vi "Main.vi"() -> ()   [LabVIEW 2010]
panel:
  out "*(type *) &x":u8
  out "unsigned 16bit integer":u16
  in  "Sample Configuration":T1(ring)
  out "Bytes Written 3":u32
  out "FT_Status 3":u32(ring) items=["FT_OK", "FT_INVALID_HANDLE", "FT_DEVICE_NOT_FOUND", "FT_DEVICE_NOT_OPENED", "FT_IO_ERROR", "FT_INSUFFICIENT_RESOURCES", "FT_INVALID_PARAMETER", "FT_INVALID_BAUD_RATE", "FT_DEVICE_NOT_OPENED_FOR_ERASE", "FT_DEVICE_NOT_OPENED_FOR_WRITE", "FT_FAILED_TO_WRITE_DEVICE", "FT_EEPROM_READ_FAILED", "FT_EEPROM_WRITE_FAILED", "FT_EEPROM_ERASE_FAILED", "FT_EEPROM_NOT_PRESENT", "FT_EEPROM_NOT_PROGRAMMED", "FT_INVALID_ARGS", "FT_NOT_SUPPORTED", "FT_OTHER_ERROR"]
  in  "Sampling Period (us)":i32=10 format="%.d"
  in  "Number of Samples":i32=1024
  in  "StopSampling":bool
  in  "StartSampling":bool
  out "XY Graph":cluster{i32[], dbl[]}[](graph)
  in  "Current Scale":enum8{"100 mA", "200 mA", "500 mA", "1 A"}(ring)
  in  "SetCurrentScale":bool
  in  "Gain":i16=700
  out "Bytes Written 2":u32
  out "FT_Status 2":u32(ring) items=["FT_OK", "FT_INVALID_HANDLE", "FT_DEVICE_NOT_FOUND", "FT_DEVICE_NOT_OPENED", "FT_IO_ERROR", "FT_INSUFFICIENT_RESOURCES", "FT_INVALID_PARAMETER", "FT_INVALID_BAUD_RATE", "FT_DEVICE_NOT_OPENED_FOR_ERASE", "FT_DEVICE_NOT_OPENED_FOR_WRITE", "FT_FAILED_TO_WRITE_DEVICE", "FT_EEPROM_READ_FAILED", "FT_EEPROM_WRITE_FAILED", "FT_EEPROM_ERASE_FAILED", "FT_EEPROM_NOT_PRESENT", "FT_EEPROM_NOT_PROGRAMMED", "FT_INVALID_ARGS", "FT_NOT_SUPPORTED", "FT_OTHER_ERROR"]
  in  "SetGain":bool
  in  "ChangeFrequency":bool
  in  "Frequency 3 (Hz)":i32=99000
  in  "Phase 3(º)":T2(ring)
  in  "Frequency 2 (Hz)":i32=99000
  in  "Phase 2 (º)":T2(ring)
  in  "Phase 1 (º)":T2(ring)
  in  "Frequency 1 (Hz)":i32=100000 format="%.d"
  out "ChB Data":i16[](array[numeric]) format="%x"
  out "ChA Data":i16[](array[numeric]) format="%x"
  out "Read Data":u8[](array[numeric]) format="%x"
  out "size(s)":i32
  out "FT_Status":u32(ring) items=["FT_OK", "FT_INVALID_HANDLE", "FT_DEVICE_NOT_FOUND", "FT_DEVICE_NOT_OPENED", "FT_IO_ERROR", "FT_INSUFFICIENT_RESOURCES", "FT_INVALID_PARAMETER", "FT_INVALID_BAUD_RATE", "FT_DEVICE_NOT_OPENED_FOR_ERASE", "FT_DEVICE_NOT_OPENED_FOR_WRITE", "FT_FAILED_TO_WRITE_DEVICE", "FT_EEPROM_READ_FAILED", "FT_EEPROM_WRITE_FAILED", "FT_EEPROM_ERASE_FAILED", "FT_EEPROM_NOT_PRESENT", "FT_EEPROM_NOT_PROGRAMMED", "FT_INVALID_ARGS", "FT_NOT_SUPPORTED", "FT_OTHER_ERROR"]
  in  "Stop Program":bool
  in  "Read":bool
  out "Bytes Waiting":u32
  out "Bytes Read":u32
  out "Description ChB":string
  out "Description ChA":string
  out "Handle ChB 2":u32
  out "Handle ChA":u32
  out "Status":bool
  in  "ChA Write Buffer":string="\u0017"
  out "Bytes Written":u32
  # "DDS Change Frequency"
  # "Set Amplification Gain"
  # "Set Probe Current Scale"
  # "Start Sampling"
  # "Configuration and Setup"
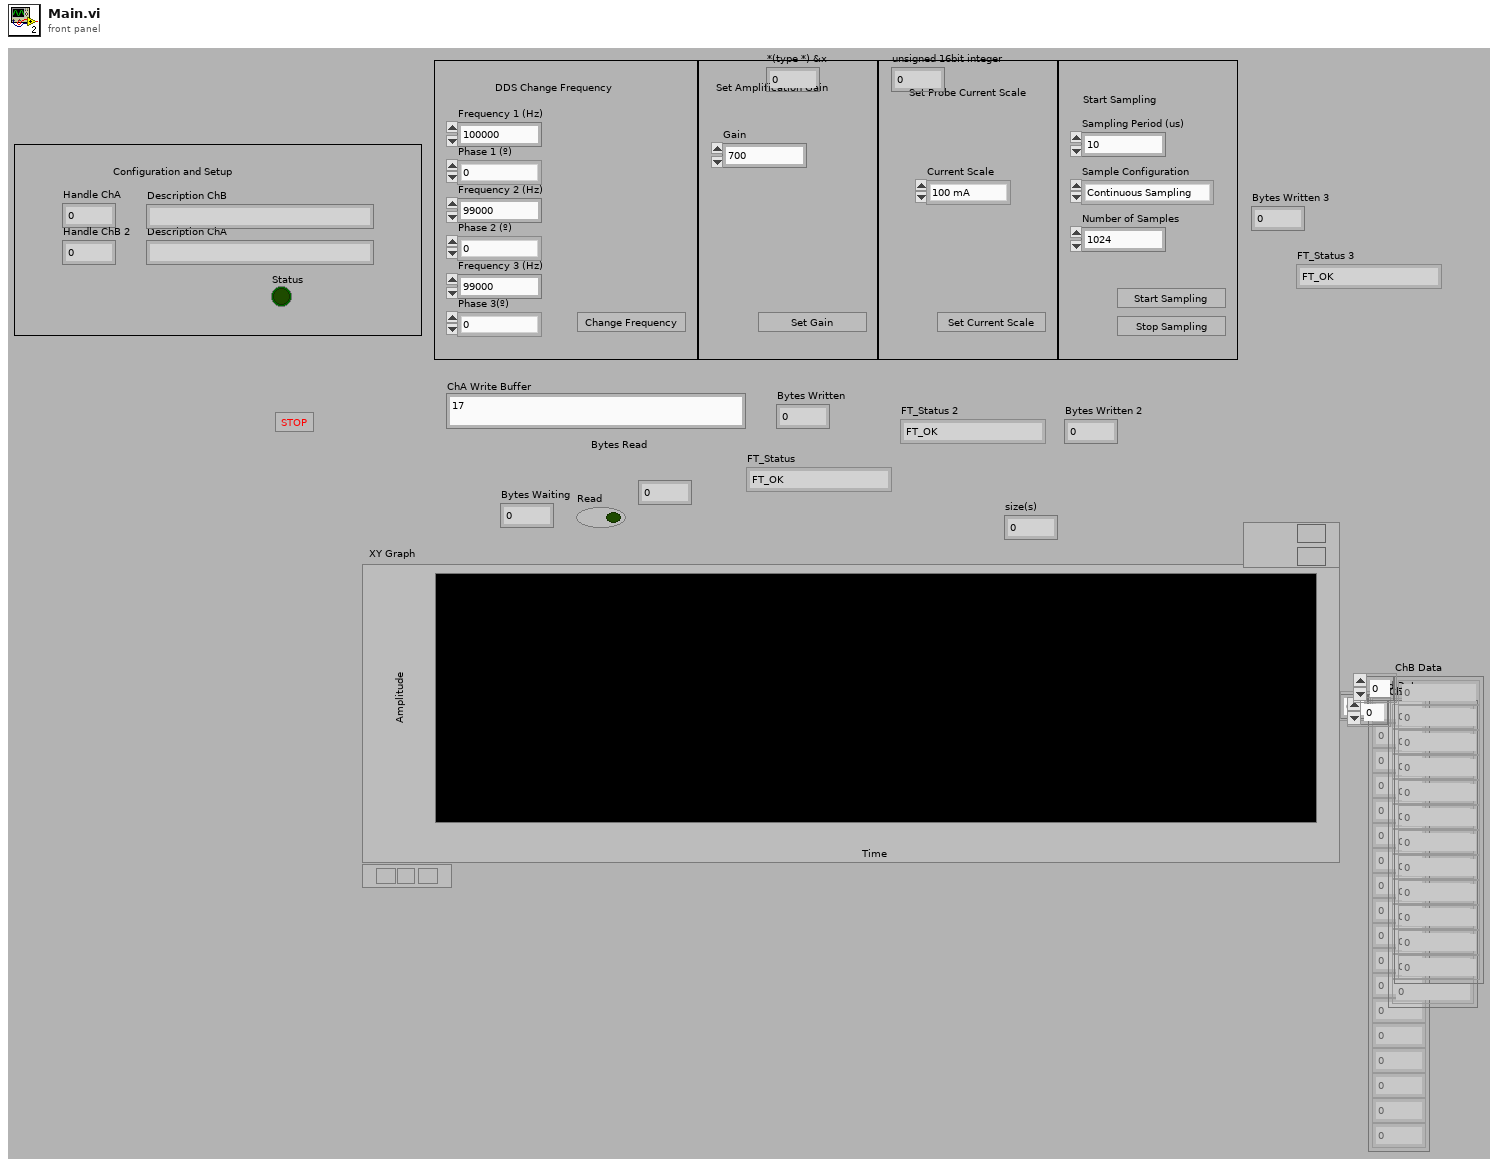
[diagram p1: front panel]
types:
  T1 = enum8{"Continuous Sampling", "Single Acquisiton"}
  T2 = enum8{"0", "11.25", "22.5", "33.75", "45", "56.25", "67.5", "78.75", "90", "101.25", "112.5", "123.75", "135", "146.25", "157.5", "168.75", "180", "191.25", "202.5", "213.75", "225", "236.25", "247.5", "258.75", "270", "281.25", "292.5", "303.75", "315", "326.25", "337.5", "348.75", "360"}
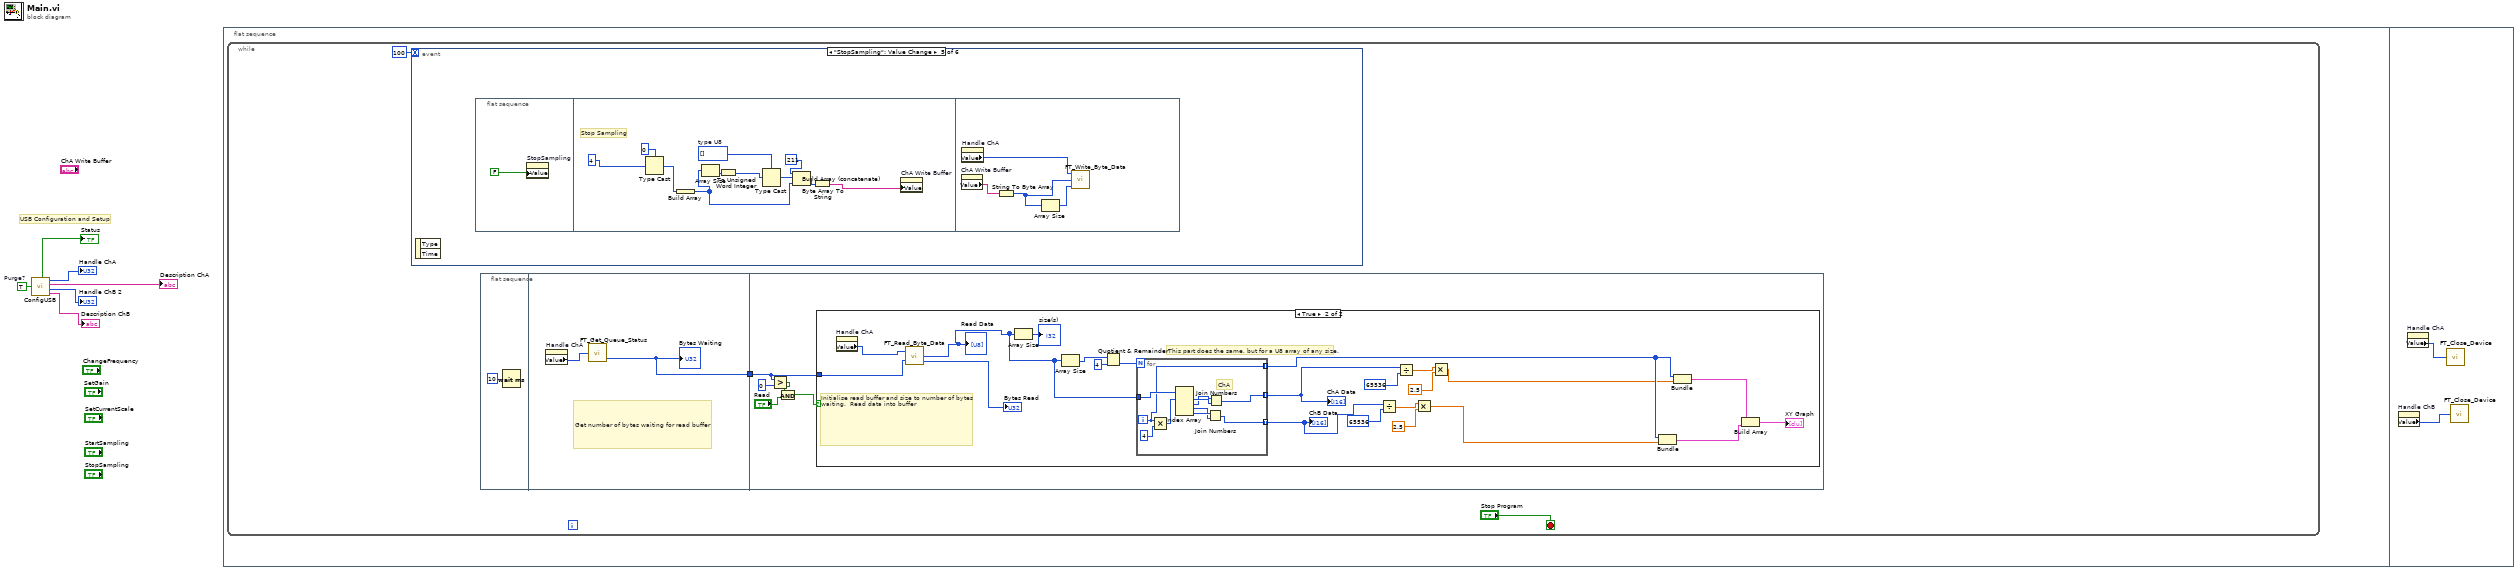
[diagram p0: block diagram]
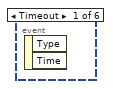
[diagram p2: hidden frame]
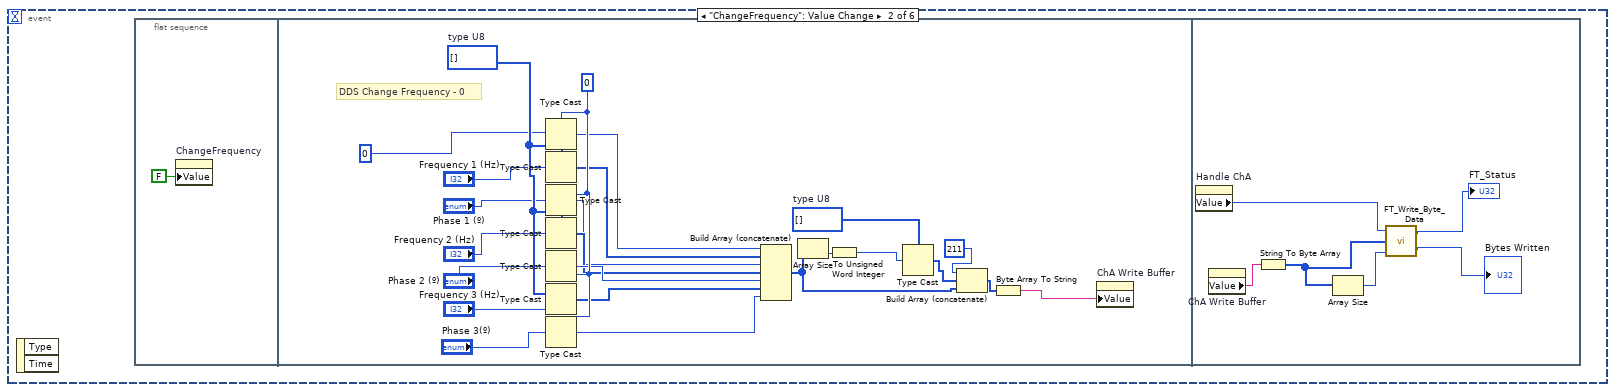
[diagram p3: hidden frame]
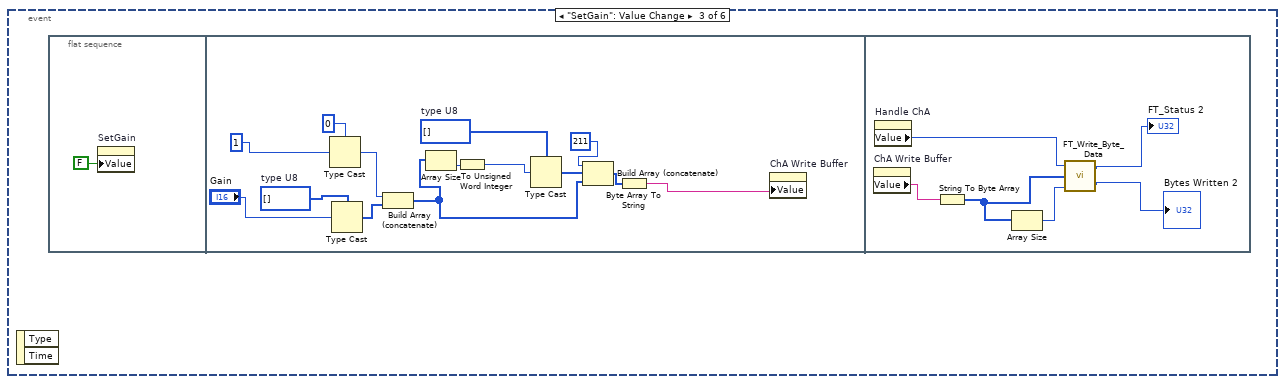
[diagram p4: hidden frame]
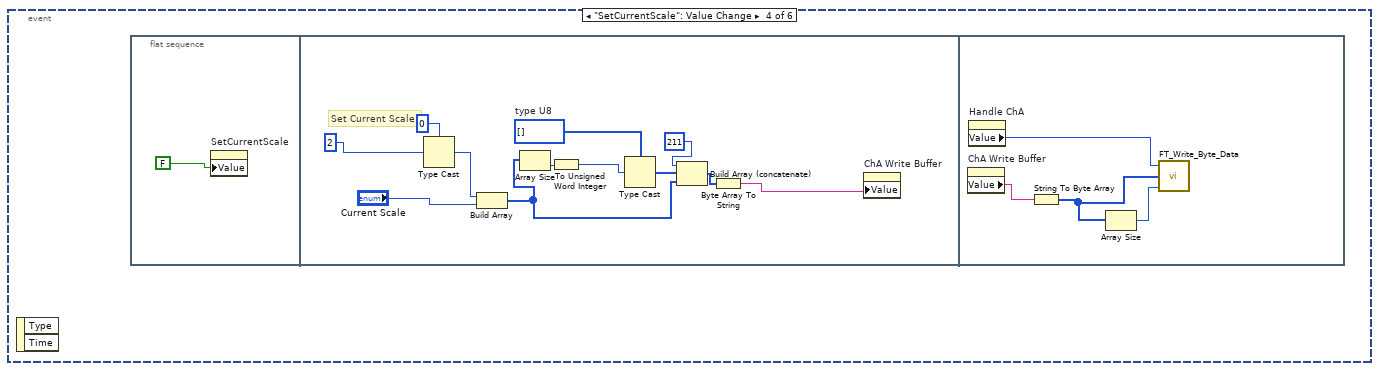
[diagram p5: hidden frame]
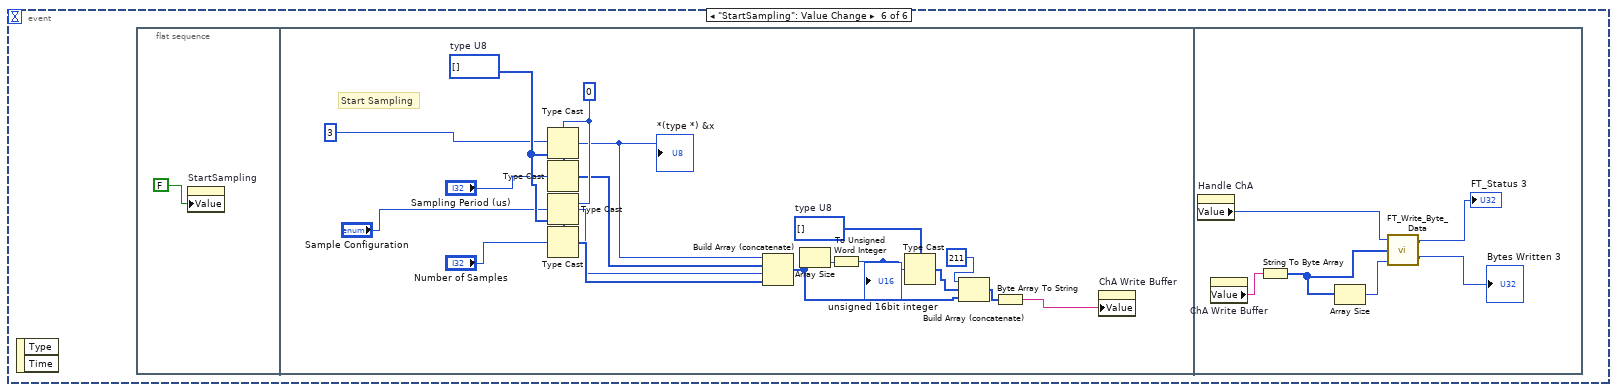
[diagram p6: hidden frame]
diagram:
  w5 = TRUE  # Purge?
  # "USB Configuration and Setup"
  n1 = call "ConfigUSB.vi"("Purge?"=w5) -> ("Status"=→"Status":bool, "Handle ChA"=→"Handle ChA":u32, "Description ChA"=→"Description ChA":string, "Handle ChB 2"=→"Handle ChB 2":u32, "Description ChB"=→"Description ChB":string)  [unwired: 5 in]
  n2 = flat-sequence {
    frame #0 {
      n3 = while {
        stop <- "Stop Program" stop-if-true
        n4 = event shown="[4] \"StopSampling\": Value Change" {
          selector: _ -> [_ _ _ _ _ _]
          dyn-events: _ -> [_ _ _ _ _ _]
          timeout: 100 -> [_ _ _ _ _ _]
          event Timeout {
            n5 = event-data() -> ()  [unwired: 1 in, 2 out]
          }
          event "ChangeFrequency": Value Change {
            n6 = event-data() -> ()  [unwired: 1 in, 2 out]
            n7 = flat-sequence {
              frame #0 {
                n8 = property on="ChangeFrequency" class="Bool (strict)"("Value"=FALSE ("ChangeFrequency")) -> ()  [unwired: 2 in, 2 out]
              }
              frame #1 {
                w32 = u8[] []  # type U8
                w29 = u8 0
                w25 = u8[] []  # type U8
                # "DDS Change Frequency - 0"
                n9 = Type Cast(type=w29, x=0) -> (*(type *) &x=w18:u8)
                n10 = Type Cast(type=w25, x="Frequency 1 (Hz)") -> (*(type *) &x=w19:u8[])
                n11 = Type Cast(type=w29, x="Phase 1 (º)") -> (*(type *) &x=w20:u8)
                n12 = Type Cast(type=w25, x="Frequency 2 (Hz)") -> (*(type *) &x=w21:u8[])
                n13 = Type Cast(type=w29, x="Phase 2 (º)") -> (*(type *) &x=w22:u8)
                n14 = Type Cast(type=w25, x="Frequency 3 (Hz)") -> (*(type *) &x=w23:u8[])
                n15 = Type Cast(type=w29, x="Phase 3(º)") -> (*(type *) &x=w24:u8)
                n16 = Build Array (concatenate)(w18, w19, w20, w21, w22, w23, w24) -> (w31:u8[])
                n17 = Array Size(array=w31) -> (size(s)=w30:i32)
                n18 = To Unsigned Word Integer(number=w30) -> (unsigned 16bit integer=w34:u16)
                n19 = Type Cast(type=w32, x=w34) -> (*(type *) &x=w33:u8[])
                n20 = Build Array (concatenate)(u8 211, w33, w31) -> (w27:u8[])
                n21 = Byte Array To String(unsigned byte array=w27) -> (string=w28:string)
                n22 = property on="ChA Write Buffer" class="Str"("Value"=w28) -> ()  [unwired: 2 in, 2 out]
              }
              frame #2 {
                n23 = property on="Handle ChA" class="DigNum (strict)"() -> ("Value"=w38:u32)  [unwired: 2 in, 2 out]
                n24 = property on="ChA Write Buffer" class="Str"() -> ("Value"=w35:string)  [unwired: 2 in, 2 out]
                n25 = String To Byte Array(string=w35) -> (unsigned byte array=w37:u8[])
                n26 = Array Size(array=w37) -> (size(s)=w36:i32)
                n27 = call "FT_Write_Byte_Data.vi"("Bytes To Write"=w36, "Buffer"=w37, "Handle"=w38) -> ("Bytes Written"=→"Bytes Written":u32, "FT_Status"=→"FT_Status":u32)
              }
            }
          }
          event "SetGain": Value Change {
            n28 = event-data() -> ()  [unwired: 1 in, 2 out]
            n29 = flat-sequence {
              frame #0 {
                n30 = property on="SetGain" class="Bool (strict)"("Value"=FALSE ("SetGain")) -> ()  [unwired: 2 in, 2 out]
              }
              frame #1 {
                w55 = u8[] []  # type U8
                w52 = u8[] []  # type U8
                n31 = Type Cast(type=u8 0, x=u8 1) -> (*(type *) &x=w44:u8)
                n32 = Type Cast(type=w55, x="Gain") -> (*(type *) &x=w45:u8[])
                n33 = Build Array (concatenate)(w44, w45) -> (w43:u8[])
                n34 = Array Size(array=w43) -> (size(s)=w53:i32)
                n35 = To Unsigned Word Integer(number=w53) -> (unsigned 16bit integer=w51:u16)
                n36 = Type Cast(type=w52, x=w51) -> (*(type *) &x=w54:u8[])
                n37 = Build Array (concatenate)(u8 211, w54, w43) -> (w49:u8[])
                n38 = Byte Array To String(unsigned byte array=w49) -> (string=w48:string)
                n39 = property on="ChA Write Buffer" class="Str"("Value"=w48) -> ()  [unwired: 2 in, 2 out]
              }
              frame #2 {
                n40 = property on="ChA Write Buffer" class="Str"() -> ("Value"=w56:string)  [unwired: 2 in, 2 out]
                n41 = property on="Handle ChA" class="DigNum (strict)"() -> ("Value"=w59:u32)  [unwired: 2 in, 2 out]
                n42 = String To Byte Array(string=w56) -> (unsigned byte array=w60:u8[])
                n43 = Array Size(array=w60) -> (size(s)=w61:i32)
                n44 = call "FT_Write_Byte_Data.vi"("Bytes To Write"=w61, "Buffer"=w60, "Handle"=w59) -> ("Bytes Written"=→"Bytes Written 2":u32, "FT_Status"=→"FT_Status 2":u32)
              }
            }
          }
          event "SetCurrentScale": Value Change {
            n45 = event-data() -> ()  [unwired: 1 in, 2 out]
            n46 = flat-sequence {
              frame #0 {
                n47 = property on="SetCurrentScale" class="Bool (strict)"("Value"=FALSE ("SetGain")) -> ()  [unwired: 2 in, 2 out]
              }
              frame #1 {
                w72 = u8[] []  # type U8
                # "Set Current Scale"
                n48 = Type Cast(type=u8 0, x=u8 2) -> (*(type *) &x=w66:u8)
                n49 = Build Array(w66, "Current Scale") -> (w65:u8[])
                n50 = Array Size(array=w65) -> (size(s)=w73:i32)
                n51 = To Unsigned Word Integer(number=w73) -> (unsigned 16bit integer=w71:u16)
                n52 = Type Cast(type=w72, x=w71) -> (*(type *) &x=w74:u8[])
                n53 = Build Array (concatenate)(u8 211, w74, w65) -> (w69:u8[])
                n54 = Byte Array To String(unsigned byte array=w69) -> (string=w68:string)
                n55 = property on="ChA Write Buffer" class="Str"("Value"=w68) -> ()  [unwired: 2 in, 2 out]
              }
              frame #2 {
                n56 = property on="ChA Write Buffer" class="Str"() -> ("Value"=w75:string)  [unwired: 2 in, 2 out]
                n57 = property on="Handle ChA" class="DigNum (strict)"() -> ("Value"=w76:u32)  [unwired: 2 in, 2 out]
                n58 = String To Byte Array(string=w75) -> (unsigned byte array=w77:u8[])
                n59 = Array Size(array=w77) -> (size(s)=w78:i32)
                n60 = call "FT_Write_Byte_Data.vi"("Bytes To Write"=w78, "Buffer"=w77, "Handle"=w76) -> ()  [unwired: 2 out]
              }
            }
          }
          event "StopSampling": Value Change {
            n61 = event-data() -> ()  [unwired: 1 in, 2 out]
            n62 = flat-sequence {
              frame #0 {
                n63 = property on="StopSampling" class="Bool (strict)"("Value"=FALSE ("SetGain")) -> ()  [unwired: 2 in, 2 out]
              }
              frame #1 {
                w88 = u8[] []  # type U8
                # "Stop Sampling"
                n64 = Type Cast(type=u8 0, x=u8 4) -> (*(type *) &x=w82:u8)
                n65 = Build Array(w82) -> (w81:u8[])
                n66 = Array Size(array=w81) -> (size(s)=w89:i32)
                n67 = To Unsigned Word Integer(number=w89) -> (unsigned 16bit integer=w87:u16)
                n68 = Type Cast(type=w88, x=w87) -> (*(type *) &x=w90:u8[])
                n69 = Build Array (concatenate)(u8 211, w90, w81) -> (w85:u8[])
                n70 = Byte Array To String(unsigned byte array=w85) -> (string=w84:string)
                n71 = property on="ChA Write Buffer" class="Str"("Value"=w84) -> ()  [unwired: 2 in, 2 out]
              }
              frame #2 {
                n72 = property on="ChA Write Buffer" class="Str"() -> ("Value"=w91:string)  [unwired: 2 in, 2 out]
                n73 = property on="Handle ChA" class="DigNum (strict)"() -> ("Value"=w92:u32)  [unwired: 2 in, 2 out]
                n74 = String To Byte Array(string=w91) -> (unsigned byte array=w93:u8[])
                n75 = Array Size(array=w93) -> (size(s)=w94:i32)
                n76 = call "FT_Write_Byte_Data.vi"("Bytes To Write"=w94, "Buffer"=w93, "Handle"=w92) -> ()  [unwired: 2 out]
              }
            }
          }
          event "StartSampling": Value Change {
            n77 = event-data() -> ()  [unwired: 1 in, 2 out]
            n78 = flat-sequence {
              frame #0 {
                n79 = property on="StartSampling" class="Bool (strict)"("Value"=FALSE ("ChangeFrequency")) -> ()  [unwired: 2 in, 2 out]
              }
              frame #1 {
                w111 = u8[] []  # type U8
                w108 = u8 0
                w104 = u8[] []  # type U8
                # "Start Sampling"
                n80 = Type Cast(type=w108, x=i8 3) -> (*(type *) &x=w100:u8)
                "*(type *) &x" <- w100
                n81 = Type Cast(type=w104, x="Sampling Period (us)") -> (*(type *) &x=w101:u8[])
                n82 = Type Cast(type=w108, x="Sample Configuration") -> (*(type *) &x=w102:u8)
                n83 = Type Cast(type=w104, x="Number of Samples") -> (*(type *) &x=w103:u8[])
                n84 = Build Array (concatenate)(w100, w101, w102, w103) -> (w110:u8[])
                n85 = Array Size(array=w110) -> (size(s)=w109:i32)
                n86 = To Unsigned Word Integer(number=w109) -> (unsigned 16bit integer=w113:u16)
                "unsigned 16bit integer" <- w113
                n87 = Type Cast(type=w111, x=w113) -> (*(type *) &x=w112:u8[])
                n88 = Build Array (concatenate)(u8 211, w112, w110) -> (w106:u8[])
                n89 = Byte Array To String(unsigned byte array=w106) -> (string=w107:string)
                n90 = property on="ChA Write Buffer" class="Str"("Value"=w107) -> ()  [unwired: 2 in, 2 out]
              }
              frame #2 {
                n91 = property on="Handle ChA" class="DigNum (strict)"() -> ("Value"=w117:u32)  [unwired: 2 in, 2 out]
                n92 = property on="ChA Write Buffer" class="Str"() -> ("Value"=w114:string)  [unwired: 2 in, 2 out]
                n93 = String To Byte Array(string=w114) -> (unsigned byte array=w116:u8[])
                n94 = Array Size(array=w116) -> (size(s)=w115:i32)
                n95 = call "FT_Write_Byte_Data.vi"("Bytes To Write"=w115, "Buffer"=w116, "Handle"=w117) -> ("Bytes Written"=→"Bytes Written 3":u32, "FT_Status"=→"FT_Status 3":u32)
              }
            }
          }
        }
        n96 = flat-sequence {
          tunnel: [w121] -> w9
          tunnel: w9 -> [w127]
          frame #0 {
            n97 = Wait (ms)(milliseconds to wait=u32 10) -> ()  [unwired: 1 out]
          }
          frame #1 {
            # "Get number of bytes waiting for read buffer"
            n98 = property on="Handle ChA" class="DigNum (strict)"() -> ("Value"=w122:u32)  [unwired: 2 in, 2 out]
            n99 = call "FT_Get_Queue_Status.vi"("Handle"=w122) -> ("Bytes Waiting"=w121:u32)  [unwired: 1 out]
            "Bytes Waiting" <- w121
          }
          frame #2 {
            n100 = Greater?(x=w127, y=u32 0) -> (0:w125:bool)
            n101 = And(x=w125, y="Read") -> (x .and. y?=w123:bool)
            n102 = case shown="True" w123 {
              tunnel: w127 -> [_ w147]
              frame False {
              }
              frame True {
                # "This part does the same, but for a U8 array of any size."
                # "Initialise read buffer and size to number of bytes waiting.  Read data into buffer"
                n103 = property on="Handle ChA" class="DigNum (strict)"() -> ("Value"=w148:u32)  [unwired: 2 in, 2 out]
                n104 = call "FT_Read_Byte_Data.vi"("Handle"=w148, "Bytes To Read"=w147) -> ("Read Data"=w142:u8[], "Bytes Read"=→"Bytes Read":u32)  [unwired: 1 out]
                "Read Data" <- w142
                n105 = Array Size(array=w142) -> (size(s)=→"size(s)":i32)
                n106 = Array Size(array=w142) -> (size(s)=w145:i32)
                n107 = Quotient & Remainder(x=w145, y=4) -> (floor(x/y)=w143:i32)  [unwired: 1 out]
                n108 = for {
                  N: w143 -> [_]
                  tunnel: w142 -> [w159]
                  tunnel: [w156] -> w134 mode=indexing
                  tunnel: [w151] -> w138 mode=indexing
                  tunnel: [w150] -> w132 mode=indexing
                  i -> [w150]
                  # "ChA"
                  n109 = Multiply(x=w150, y=4) -> (x*y=w157:i32)
                  n110 = Index Array(array=w159, index #1=w157) -> (element #1=w155:u8, element #2=w154:u8, element #3=w152:u8, element #4=w153:u8)  [unwired: 3 in]
                  n111 = Join Numbers(hi=w153, lo=w152) -> ((hi.lo)=w151:u16)
                  n112 = Join Numbers(hi=w154, lo=w155) -> ((hi.lo)=w156:u16)
                }
                "ChA Data" <- w134
                "ChB Data" <- w138
                n113 = Divide(x=w138, y=65536) -> (x/y=w140:dbl[])
                n114 = Divide(x=w134, y=65536) -> (x/y=w136:dbl[])
                n115 = Multiply(x=w140, y=2.5) -> (x*y=w130:dbl[])
                n116 = Multiply(x=w136, y=2.5) -> (x*y=w131:dbl[])
                n117 = Bundle(w132, w130) -> (w129:cluster{i32[], dbl[]})  [unwired: 1 in]
                n118 = Bundle(w132, w131) -> (w133:cluster{i32[], dbl[]})  [unwired: 1 in]
                n119 = Build Array(w133, w129) -> (→"XY Graph":cluster{i32[], dbl[]}[])
              }
            }
          }
        }
      }
    }
    frame #1 {
      n120 = property on="Handle ChB" class="DigNum (strict)"() -> ("Value"=w160:u32)  [unwired: 2 in, 2 out]
      n121 = property on="Handle ChA" class="DigNum (strict)"() -> ("Value"=w161:u32)  [unwired: 2 in, 2 out]
      n122 = call "FT_Close_Device.vi"("Handle"=w161) -> ()  [unwired: 1 out]
      n123 = call "FT_Close_Device.vi"("Handle"=w160) -> ()  [unwired: 1 out]
    }
  }
